vi "AddChangeData(SubVI).vi"(6 "String in":string, 8 "Error In":errorcluster, 9 "XYGraph Refnum":refnum<vi>, 10 "Arr Refnum":refnum<vi>, 11 "ComboBox in":refnum<vi>) -> (0 "Error Out":errorcluster)   [LabVIEW 2018]
uses:
  CTL/Line.ctl
  Windows/Settings/View.ctl
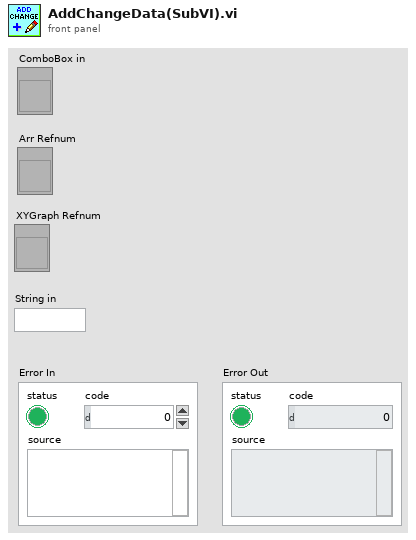
[diagram p1: front panel]
types:
  T1 = typedef "Line.ctl" = cluster{"Width":dbl, "Color":i64, "Array Oy":dbl[], "Array Ox":dbl[], "Name":string, "Plot Visible":T2}
  T2 = typedef "View.ctl" = bool
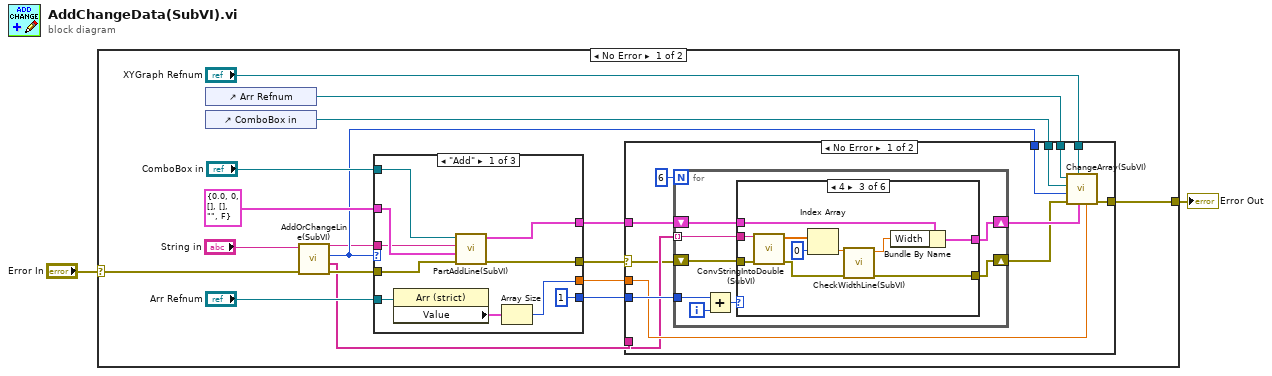
[diagram p0: block diagram]
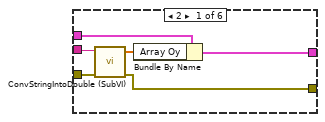
[diagram p2: hidden frame]
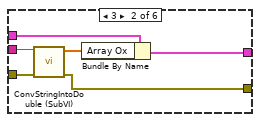
[diagram p3: hidden frame]
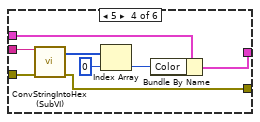
[diagram p4: hidden frame]
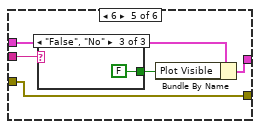
[diagram p5: hidden frame]
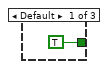
[diagram p6: hidden frame]
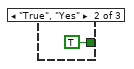
[diagram p7: hidden frame]
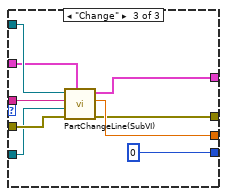
[diagram p11: hidden frame]
diagram:
  n1 = case shown="No Error" "Error In" {
    selector: "Error In" -> [w12 w102]
    tunnel: [w10 w102] -> w1
    frame No Error {
      n2 = control-ref of="Arr Refnum"() -> (w16:refnum<vi>)
      n3 = control-ref of="ComboBox in"() -> (w14:refnum<vi>)
      n4 = call "AddOrChangeLine(SubVI).vi"("error in (no error)"=w12, "String in"="String in") -> ("error out"=w11:errorcluster, "String Array Out"=w7:string[], "Enum"=w5:enum16{"Default", "Change", "Add"}, "String out"=w3:string)  [unwired: 6 in]
      n5 = case shown="\"Add\"" w5 {
        tunnel: [w91 _ w101] -> w18
        tunnel: T1 {"Width"=0.0, "Color"=0, "Array Oy"=[], "Array Ox"=[], "Name"="", "Plot Visible"=FALSE} ("element") -> [w85 _ w95]
        tunnel: [1 ("x") _ 0 ("x")] -> w17
        tunnel: [w89 _ w99] -> w13
        tunnel: w11 -> [w88 w92 w98]
        tunnel: [w87 w92 w97] -> w6
        tunnel: "ComboBox in" -> [w86 _ w96]
        tunnel: "Arr Refnum" -> [w84 _ w94]
        tunnel: w3 -> [w82 _ w93]
        frame "Add" {
          n6 = property class="Arr (strict)"(reference=w84) -> ("Value"=w83:T1[])  [unwired: 1 in, 2 out]
          n7 = call "PartAddLine(SubVI).vi"("error in (no error)"=w88, "element in"=w85, "String in"=w82, "ComboBox in"=w86) -> ("error out"=w87:errorcluster, "element out"=w91:T1)  [unwired: 6 in]
          n8 = Array Size(array=w83) -> (size(s)=w89:i32)
        }
        frame "Default" {
        }
        frame "Change" {
          n9 = call "PartChangeLine(SubVI).vi"("element in"=w95, "error in (no error)"=w98, "Arr Refnum"=w94, "String in"=w93, "ComboBox in"=w96) -> ("error out"=w97:errorcluster, "NumPlot"=w99:dbl, "element out"=w101:T1)  [unwired: 4 in]
        }
      }
      n10 = case shown="No Error" w6 {
        selector: w6 -> [w21 w81]
        tunnel: w18 -> [w31 _]
        tunnel: w17 -> [w30 _]
        tunnel: w16 -> [w29 _]
        tunnel: "XYGraph Refnum" -> [w28 _]
        tunnel: w14 -> [w27 _]
        tunnel: w13 -> [w26 _]
        tunnel: [w24 w81] -> w10
        tunnel: w7 -> [w23 _]
        tunnel: w5 -> [w20 _]
        frame No Error {
          n11 = for {
            N: 6 -> [_]
            shift-right: [w40] -> w25
            shift-left: w31 -> [w39]
            tunnel: w30 -> [w36]
            tunnel: w23 -> [w35] mode=indexing
            shift-right: [w33] -> w22
            shift-left: w21 -> [w34]
            i -> [w37]
            n12 = Add(x=w36, y=w37) -> (x+y=w38:i32)
            n13 = case shown="4" w38 {
              tunnel: [w45 w52 w58 w67 w74 w80] -> w40
              tunnel: w39 -> [w44 w50 w57 w66 w73 w80]
              tunnel: w34 -> [w43 w49 w56 w65 w72 w79]
              tunnel: [w42 w48 w53 w64 w72 w79] -> w33
              tunnel: w35 -> [w41 w47 w55 w63 w71 _]
              frame 2 {
                n14 = call "ConvStringIntoDouble (SubVI).vi"("Error In"=w43, "String In"=w41) -> ("Error Out"=w42:errorcluster, "Array Out"=w46:dbl[])  [unwired: 6 in]
                n15 = Bundle By Name(cluster=w44, "Array Oy"=w46) -> (w45:T1)
              }
              frame 3 {
                n16 = call "ConvStringIntoDouble (SubVI).vi"("Error In"=w49, "String In"=w47) -> ("Error Out"=w48:errorcluster, "Array Out"=w51:dbl[])  [unwired: 6 in]
                n17 = Bundle By Name(cluster=w50, "Array Ox"=w51) -> (w52:T1)
              }
              frame 4 {
                n18 = call "ConvStringIntoDouble (SubVI).vi"("Error In"=w56, "String In"=w55) -> ("Error Out"=w54:errorcluster, "Array Out"=w62:dbl[])  [unwired: 6 in]
                n19 = Index Array(array=w62, index=0) -> (element=w60:dbl)
                n20 = call "CheckWidthLine(SubVI).vi"("Error In"=w54, "Input"=w60) -> ("Error Out"=w53:errorcluster, "Output"=w59:dbl)  [unwired: 8 in]
                n21 = Bundle By Name(cluster=w57, "Width"=w59) -> (w58:T1)
              }
              frame 5 {
                n22 = call "ConvStringIntoHex (SubVI).vi"("Error In"=w65, "String In"=w63) -> ("Error Out"=w64:errorcluster, "Array Out"=w70:i64[])  [unwired: 8 in]
                n23 = Index Array(array=w70, index=0) -> (element=w68:i64)
                n24 = Bundle By Name(cluster=w66, "Color"=w68) -> (w67:T1)
              }
              frame 6 {
                n25 = case shown="\"False\", \"No\"" w71 {
                  tunnel: [TRUE TRUE FALSE] -> w75
                  frame Default {
                  }
                  frame "True", "Yes" {
                  }
                  frame "False", "No" {
                  }
                }
                n26 = Bundle By Name(cluster=w73, "Plot Visible"=w75) -> (w74:T1)
              }
              frame Default {
              }
            }
          }
          n27 = call "ChangeArray(SubVI).vi"("NumPlot"=w26, "element"=w25, "XYGraph Refnum"=w28, "Error In"=w22, "Enum"=w20, "ComboBox in"=w27, "LVObjectRefNum in"=w29) -> ("Error Out"=w24:errorcluster)  [unwired: 4 in]
        }
        frame Error {
        }
      }
    }
    frame Error {
    }
  }
  "Error Out" <- w1
